vi "Sub_Create_Remaining_Length.vi"(8 "error in (no error)":errorcluster, 11 "X":u32) -> (0 "error out":errorcluster, 3 "bytes":u8[](array[numeric]) format="%x")   [LabVIEW 2019, in "MQTT_Functions.lvlib"]
uses:
  MQTT_Functions.lvlib
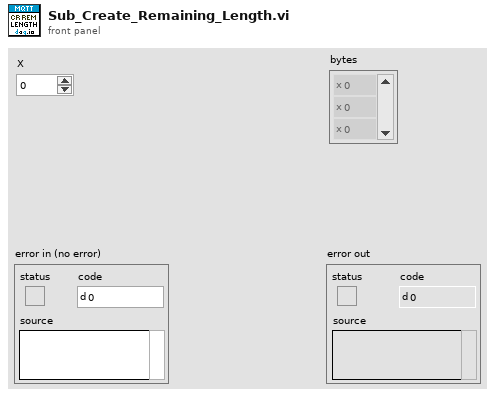
[diagram p1: front panel]
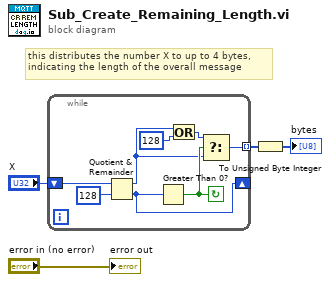
[diagram p0: block diagram]
diagram:
  # "this distributes the number X to up to 4 bytes, \nindicating the length of the overall message"
  n1 = while {
    shift-right: [w6] -> _
    shift-left: "X" -> [w10]
    tunnel: [w8] -> w4 mode=indexing
    stop <- w9 continue-if-true
    n2 = Quotient & Remainder(x=w10, y=u32 128) -> (x-y*floor(x/y)=w5:u32, floor(x/y)=w6:u32)
    n3 = Greater Than 0?(x=w6) -> (x > 0?=w9:bool)
    n4 = Or(x=w5, y=u32 128) -> (x .or. y?=w7:u32)
    n5 = Select(t=w7, s=w9, f=w5) -> (s? t:f=w8:u32)
  }
  n6 = To Unsigned Byte Integer(number=w4) -> (unsigned 8bit integer=→"bytes":u8[])
  "error out" <- "error in (no error)"
